vi "Fake ADC.vi"(8 "error in (no error)":errorcluster, 11 "AI select":dbl) -> (0 "error out":errorcluster, 3 "Ouptut":dbl)   [LabVIEW 2013]
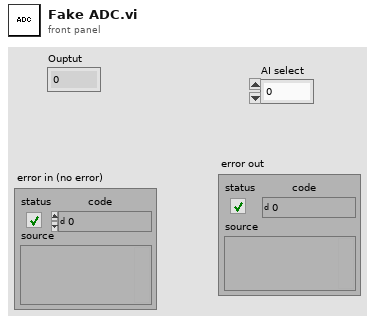
[diagram p1: front panel]
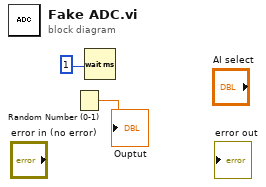
[diagram p0: block diagram]
diagram:
  n1 = Random Number (0-1)() -> (number: 0 to 1=→"Ouptut":dbl)
  n2 = Wait (ms)(milliseconds to wait=u32 1) -> ()  [unwired: 1 out]
